vi "GEA2 Read ERD.vi"(0 "GEA2 Reference In":refnum<k24>, 1 "Retry Count":i32=2 step=1, 2 "Read Timeout (ms)":u32=500, 5 "GEA Inputs":T2 {"Destination" format="%.0x"; "Source" format="%.0x"}, 7 "Read ERD List":T3[](array[typedef]) {"ERD Number" format="%.0x"}, 11 "Error In":errorcluster, 12 "Low Level Tries":u8=5 min=1, 13 "Verify ERD Response?":bool=TRUE) -> (4 "GEA2 Reference Out":refnum<k24>, 6 "Raw Data Out":string, 8 "ERD Data Out":T1[](array[typedef]) {"ERD Number" format="%.0x"}, 15 "Error Out":errorcluster)   [LabVIEW 2023, in "GEA2_Toolkit.lvlib"]
doc: "This VI reads an array of ERDs with a single command and returns the data in the data type selected."
uses:
  GEA3/library/GEA2_Toolkit.lvlib
  D:/Common/LabVIEW GEA2 Toolkit/source/GEA3 DLL Source/GeaCommunication.dll
  source/GEA3 DLL Source/GeaCommunication.dll
  GEA3/type defs/ERD Read Data In.ctl
  GEA3/type defs/Source_Destination.ctl
  GEA3/type defs/ERD Read Data Out.ctl
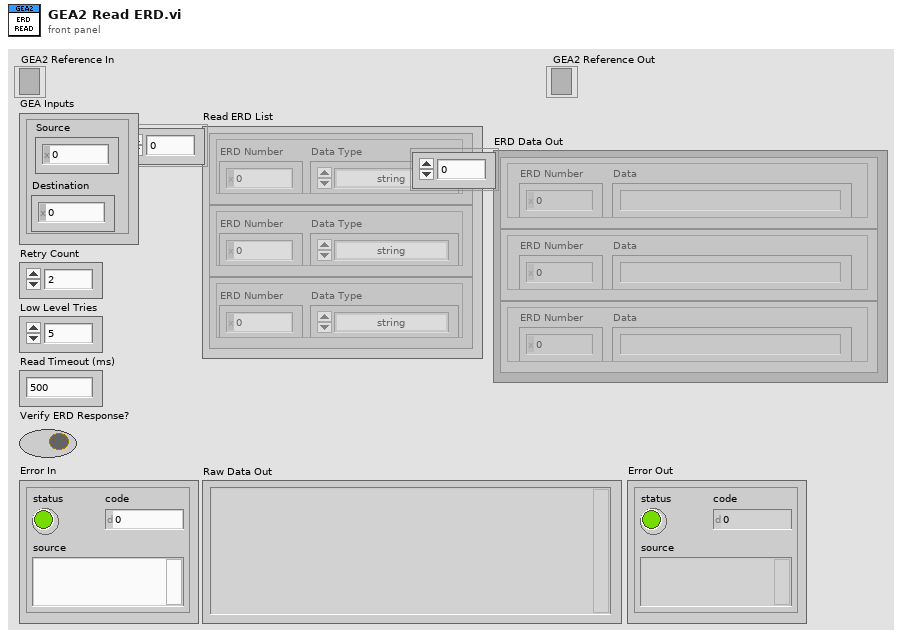
[diagram p1: front panel]
types:
  T1 = typedef "ERD Read Data Out.ctl" = cluster{"ERD Number":u16, "Data":string}
  T2 = typedef "Source_Destination.ctl" = cluster{"Source":u8, "Destination":u8}
  T3 = typedef "ERD Read Data In.ctl" = cluster{"ERD Number":u16, "Data Type":enum16{"string", "boolean", "uint8_t", "uint16_t", "uint32_t", "uint64_t", "int8_t", "int16_t", "int32_t", "int64_t"}}
  T4 = typedef "Data In.ctl" = cluster{"Source":u8, "Destination":u8, "Command":u8, "Message":string}
  T5 = typedef "GEA2_Toolkit.lvlib/Data Out.ctl" = cluster{"Source":u8, "Destination":u8, "Command":u8, "Length":u8, "CRC":u16, "Message":string}
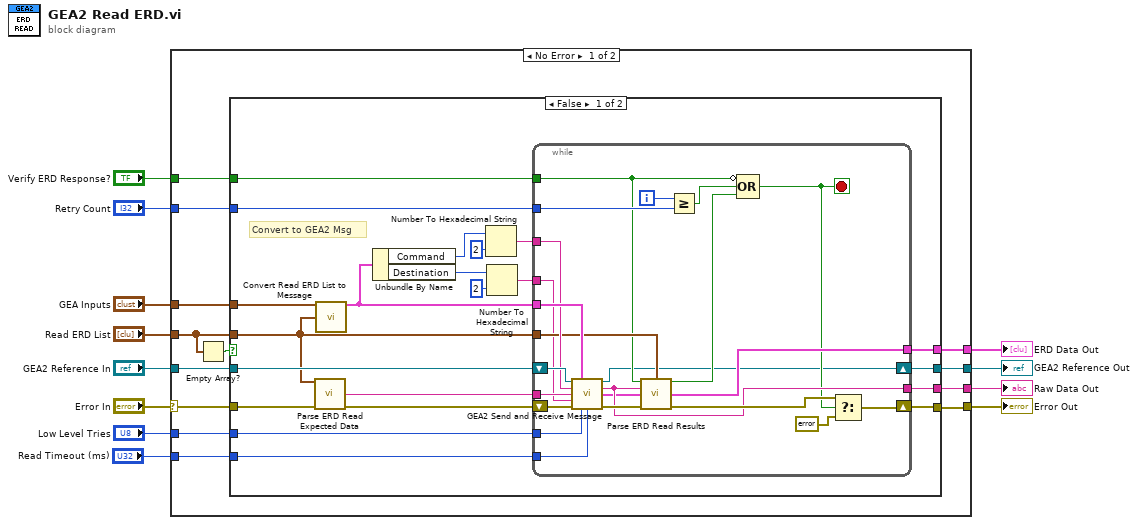
[diagram p0: block diagram]
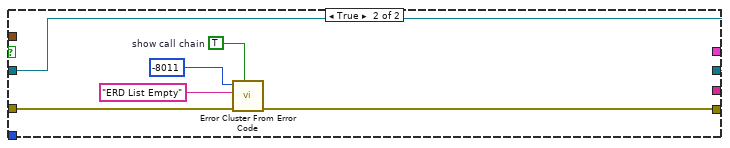
[diagram p2: hidden frame]
diagram:
  n1 = case shown="No Error" "Error In" {
    selector: "Error In" -> [w25 w76]
    tunnel: "GEA2 Reference In" -> [w24 w77]
    tunnel: "Read ERD List" -> [w15 _]
    tunnel: "Verify ERD Response?" -> [w22 _]
    tunnel: "GEA Inputs" -> [w23 _]
    tunnel: [w18 _] -> w8
    tunnel: [w19 w76] -> w2
    tunnel: "Read Timeout (ms)" -> [w21 _]
    tunnel: "Retry Count" -> [w20 _]
    tunnel: [w17 w77] -> w5
    tunnel: [w16 _] -> w4
    tunnel: "Low Level Tries" -> [w13 _]
    frame No Error {
      n2 = Empty Array?(array=w15) -> (empty?=w14:bool)
      n3 = case shown="False" w14 {
        tunnel: w25 -> [w40 w72]
        tunnel: w24 -> [w46 w70]
        tunnel: w23 -> [w45 _]
        tunnel: w22 -> [w44 _]
        tunnel: w21 -> [w43 _]
        tunnel: w20 -> [w42 _]
        tunnel: [w30 w71] -> w19
        tunnel: [w31 _] -> w18
        tunnel: [w29 w70] -> w17
        tunnel: [w32 _] -> w16
        tunnel: w15 -> [w41 _]
        tunnel: w13 -> [w33 _]
        frame False {
          # "Convert to GEA2 Msg"
          n4 = call "Parse ERD Read Expected Data.vi"("Read ERD List"=w41, "Error In"=w40) -> ("Expected Data"=w39:string, "Error Out"=w38:errorcluster)  [unwired: 12 in]
          n5 = call "Convert Read ERD List to Message.vi"("GEA Inputs"=w45, "Read ERD List"=w41) -> ("GEA Message"=w36:T4)  [unwired: 12 in, 1 out]
          n6 = Unbundle By Name(w36) -> ("Command"=w35:u8, "Destination"=w27:u8)
          n7 = Number To Hexadecimal String(1:i16 2 ("width (-)"), 2:w35) -> (0:w34:string)
          n8 = Number To Hexadecimal String(1:i16 2 ("width (-)"), 2:w27) -> (0:w26:string)
          n9 = while {
            tunnel: w36 -> [w60]
            tunnel: [w52] -> w31
            tunnel: w44 -> [w50]
            tunnel: w41 -> [w53]
            tunnel: [w65] -> w32
            tunnel: w43 -> [w69]
            tunnel: w42 -> [w67]
            tunnel: w39 -> [w62]
            shift-right: [w54] -> w30
            shift-left: w38 -> [w61]
            shift-right: [w48] -> w29
            shift-left: w46 -> [w66]
            tunnel: w34 -> [w59]
            tunnel: w33 -> [w58]
            tunnel: w26 -> [w47]
            i -> [w68]
            stop <- w49 stop-if-true
            n10 = call "GEA2 Send and Receive Message.vi"("GEA2 Reference In"=w66, "Input Data"=w60, "Read Timeout (ms)"=w69, "Expected Command"=w59, "Expected Data"=w62, "Expected Source"=w47, "Error In"=w61, "# of Tries"=w58) -> ("GEA2 Reference Out"=w48:refnum<k24>, "Raw Data Out"=w52:string, "Converted Data Out"=w51:T5, "Error Out"=w57:errorcluster)  [unwired: 4 in]
            n11 = call "Parse ERD Read Results.vi"("Verify ERD Response?"=w50, "Read ERD List"=w53, "Raw Message"=w52, "Converted Data"=w51, "Error In"=w57) -> ("Pass/Fail?"=w63:bool, "ERD Data Out"=w65:T1[], "Error Out"=w56:errorcluster)  [unwired: 8 in]
            n12 = Greater Or Equal?(x=w68, y=w67) -> (x >= y?=w64:bool)
            n13 = Compound Arithmetic op=OR(invert w50, w64, w63) -> (w49:bool)
            n14 = Select(t=w56, s=w49, f=errorcluster {"status"=FALSE, "code"=0, "source"=""}) -> (s? t:f=w54:errorcluster)
          }
        }
        frame True {
          w73 = TRUE  # show call chain
          n15 = call <vilib>:"Error Cluster From Error Code.vi"("show call chain? (False)"=w73, "error in (no error)"=w72, "error message (\"\")"="ERD List Empty" ("error message (\"\")"), "error code (0)"=-8011) -> ("error out"=w71:errorcluster)  [unwired: 5 in]
        }
      }
    }
    frame Error {
    }
  }
  "Raw Data Out" <- w8
  "GEA2 Reference Out" <- w5
  "ERD Data Out" <- w4
  "Error Out" <- w2
